vi "MQTT_Connect.vi"(5 "Connect Meta":T5={"QoS"=enum."At most once", "DUP"=FALSE, "Retain"=TRUE, "Keep Alive (sec)"=60}, 6 "Client ID":string="LabVIEW_MQTT_Client", 7 "Connect Flags":T8, 8 "error in (no error)":errorcluster, 9 "Will Info":T6={"Will message"="Last Will", "Will Topic"="Will Topic"}, 10 "User Info":T7={"User Name"="User", "Password"="password"}, 11 "MQTT Broker":cluster{"address (IP)":string, "port":u16}={"address (IP)"="broker.mqttdashboard.com", "port"=1883}) -> (0 "error out":errorcluster, 2 "Connection Status":T1=enum."Connection refused: not authorized", 3 "connection ID out":refnum<k5>)   [LabVIEW 2025, in "MQTT_Functions.lvlib"]
doc: "Connects to an MQTT broker server with required settings. \n\n© 2015 - daq.io, LLC - Peter Adelhardt"
uses:
  MQTT_Functions.lvlib
  Controls/Connect_Flags.ctl
  Controls/QoS.ctl
  Controls/User_Info.ctl
  Controls/Will_Info.ctl
  Controls/DUP_Flag.ctl
  Controls/Retain_Flag.ctl
  Controls/Connection_Return_Codes.ctl
  Controls/Conn_FGV_Cmds.ctl
  Controls/Conn_Stat_FGV_Cmds.ctl
  Controls/MessageType.ctl
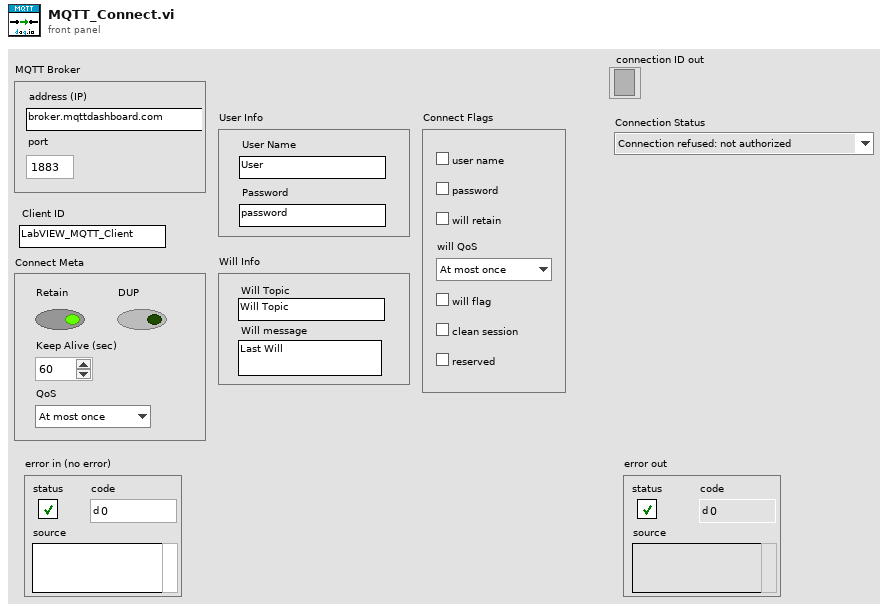
[diagram p1: front panel]
types:
  T1 = typedef "MQTT_Functions.lvlib/Connection_Return_Codes.ctl" = enum16{"Connection accepted", "Connection refused: unacceptable protocol version", "Connection refused: identifier rejected", "Connection refused: Server unavailable", "Connection refused: bad user name or password", "Connection refused: not authorized"}
  T2 = typedef "MQTT_Functions.lvlib/QoS.ctl" = enum8{"At most once", "At least once", "Exactly once", "Reserved"}
  T3 = typedef "MQTT_Functions.lvlib/DUP_Flag.ctl" = bool
  T4 = typedef "MQTT_Functions.lvlib/Retain_Flag.ctl" = bool
  T5 = cluster{"QoS":T2, "DUP":T3, "Retain":T4, "Keep Alive (sec)":u16}
  T6 = typedef "MQTT_Functions.lvlib/Will_Info.ctl" = cluster{"Will message":string, "Will Topic":string}
  T7 = typedef "MQTT_Functions.lvlib/User_Info.ctl" = cluster{"User Name":string, "Password":string}
  T8 = typedef "MQTT_Functions.lvlib/Connect_Flags.ctl" = cluster{"user name":bool, "password":bool, "will retain":bool, "will flag":bool, "clean session":bool, "reserved":bool, "will QoS":T2}
  T9 = typedef "MQTT_Functions.lvlib/Conn_Stat_FGV_Cmds.ctl" = enum16{"Get", "Set"}
  T10 = typedef "MQTT_Functions.lvlib/Conn_FGV_Cmds.ctl" = enum16{"Get", "Set", "Delete"}
  T11 = typedef "MQTT_Functions.lvlib/MessageType.ctl" = enum32{"Reserved", "CONNECT", "CONNACK", "PUBLISH", "PUBACK", "PUBREC", "PUBREL", "PUBCOMP", "SUBSCRIBE", "SUBACK", "UNSUBSCRIBE", "UNSUBACK", "PINGREQ", "PINGRESP", "DISCONNECT", "Reserved2"}
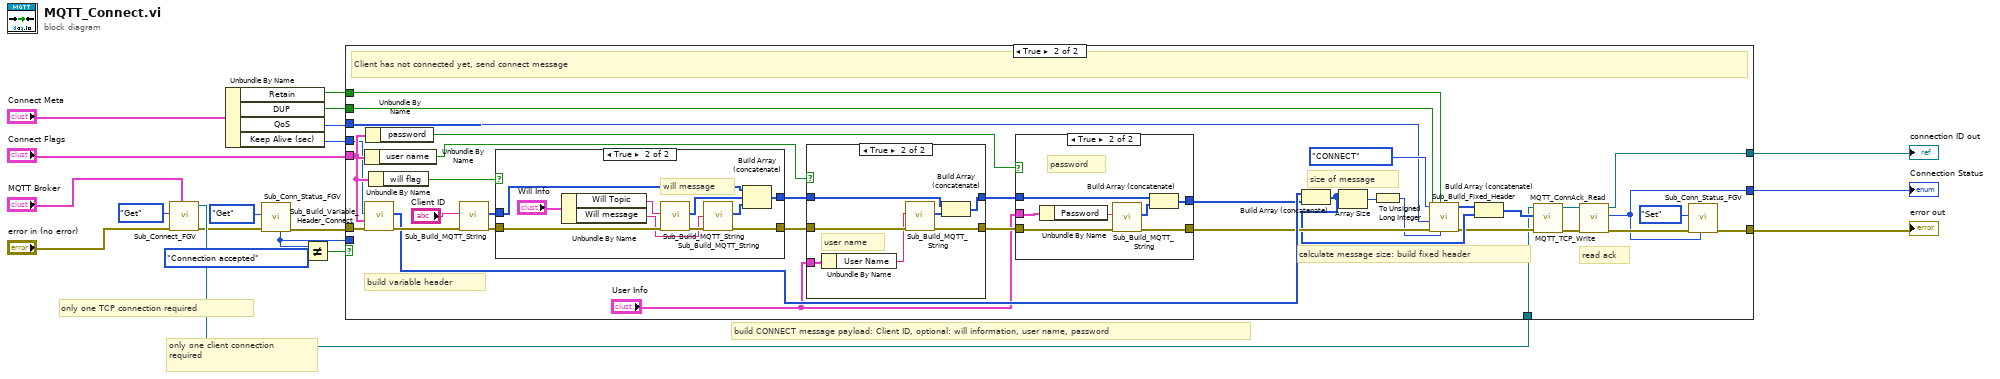
[diagram p0: block diagram]
diagram:
  # "only one client connection\nrequired"
  # "only one TCP connection required"
  # "build CONNECT message payload: Client ID, optional: will information, user name, password"
  n1 = call "Sub_Connect_FGV.vi"("MQTT Broker"="MQTT Broker", "error in"="error in (no error)", "Command"=Conn_FGV_Cmds."Get") -> ("error out"=w5:errorcluster, "MQTT ref out"=w12:refnum<k5>)  [unwired: 7 in]
  n2 = Unbundle By Name("Connect Meta") -> ("Retain"=w17:T4, "DUP"=w16:T3, "QoS"=w15:T2, "Keep Alive (sec)"=w14:u16)
  n3 = call "Sub_Conn_Status_FGV.vi"("error in"=w5, "Command"=Conn_Stat_FGV_Cmds."Get") -> ("error out"=w2:errorcluster, "Connection Status out"=w1:T1)  [unwired: 8 in]
  n4 = Not Equal?(x=w1, y=Connection_Return_Codes."Connection accepted") -> (x != y?=w3:bool)
  n5 = case shown="True" w3 {
    tunnel: "Connect Flags" -> [_ w52]
    tunnel: w17 -> [_ w38]
    tunnel: w16 -> [_ w37]
    tunnel: w15 -> [_ w36]
    tunnel: w14 -> [_ w35]
    tunnel: w2 -> [w22 w29]
    tunnel: w12 -> [w20 w28]
    tunnel: [w22 w24] -> w9
    tunnel: [w21 w23] -> w8
    tunnel: [w20 w27] -> w7
    tunnel: w1 -> [w21 _]
    frame False {
      # "client is already connected"
    }
    frame True {
      # "read ack"
      # "calculate message size: build fixed header"
      # "build variable header"
      # "size of message"
      # "Client has not connected yet, send connect message"
      n6 = Unbundle By Name(w52) -> ("user name"=w51:bool)
      n7 = call "Sub_Build_Variable_Header_Connect.vi"("error in (no error)"=w29, "Connect Flags"=w52, "Keep Alive (sec)"=w35) -> ("error out"=w57:errorcluster, "Variable Header"=w48:u8[])  [unwired: 7 in]
      n8 = Unbundle By Name(w52) -> ("password"=w50:bool)
      n9 = Unbundle By Name(w52) -> ("will flag"=w49:bool)
      n10 = call "Sub_Build_MQTT_String.vi"("error in (no error)"=w57, "String to be encoded"="Client ID") -> ("error out"=w53:errorcluster, "UTF8 Byte Array"=w56:u8[])  [unwired: 8 in]
      n11 = case shown="True" w49 {
        tunnel: w56 -> [w78 w86]
        tunnel: [w78 w87] -> w55
        tunnel: w53 -> [w77 w85]
        tunnel: [w77 w82] -> w46
        frame False {
        }
        frame True {
          # "will message"
          n12 = Unbundle By Name("Will Info") -> ("Will Topic"=w80:string, "Will message"=w79:string)
          n13 = call "Sub_Build_MQTT_String.vi"("error in (no error)"=w85, "String to be encoded"=w80) -> ("error out"=w84:errorcluster, "UTF8 Byte Array"=w83:u8[])  [unwired: 8 in]
          n14 = call "Sub_Build_MQTT_String.vi"("error in (no error)"=w84, "String to be encoded"=w79) -> ("error out"=w82:errorcluster, "UTF8 Byte Array"=w88:u8[])  [unwired: 8 in]
          n15 = Build Array (concatenate)(w86, w83, w88) -> (w87:u8[])
        }
      }
      n16 = case shown="True" w51 {
        tunnel: w55 -> [w69 w75]
        tunnel: [w69 w74] -> w54
        tunnel: [w68 w73] -> w47
        tunnel: w46 -> [w68 w72]
        tunnel: "User Info" -> [_ w71]
        frame False {
        }
        frame True {
          # "user name"
          n17 = Unbundle By Name(w71) -> ("User Name"=w70:string)
          n18 = call "Sub_Build_MQTT_String.vi"("error in (no error)"=w72, "String to be encoded"=w70) -> ("error out"=w73:errorcluster, "UTF8 Byte Array"=w76:u8[])  [unwired: 8 in]
          n19 = Build Array (concatenate)(w75, w76) -> (w74:u8[])
        }
      }
      n20 = case shown="True" w50 {
        tunnel: w54 -> [w60 w66]
        tunnel: [w60 w65] -> w44
        tunnel: w47 -> [w59 w64]
        tunnel: [w59 w63] -> w45
        tunnel: "User Info" -> [_ w62]
        frame False {
        }
        frame True {
          # "password"
          n21 = Unbundle By Name(w62) -> ("Password"=w61:string)
          n22 = call "Sub_Build_MQTT_String.vi"("error in (no error)"=w64, "String to be encoded"=w61) -> ("error out"=w63:errorcluster, "UTF8 Byte Array"=w67:u8[])  [unwired: 8 in]
          n23 = Build Array (concatenate)(w66, w67) -> (w65:u8[])
        }
      }
      n24 = Build Array (concatenate)(w48, w44) -> (w43:u8[])
      n25 = Array Size(array=w43) -> (size(s)=w41:i32)
      n26 = To Unsigned Long Integer(number=w41) -> (unsigned 32bit integer=w40:u32)
      n27 = call "Sub_Build_Fixed_Header.vi"("Remaining Length"=w40, "Retain"=w38, "error in (no error)"=w45, "QoS"=w36, "DUP"=w37, "MessageType"=MessageType."CONNECT") -> ("error out"=w33:errorcluster, "Fixed Header"=w42:u8[])  [unwired: 4 in]
      n28 = Build Array (concatenate)(w42, w43) -> (w32:u8[])
      n29 = call "MQTT_TCP_Write.vi"("error in (no error)"=w33, "data in"=w32, "connection ID"=w28) -> ("error out"=w31:errorcluster, "connection ID out"=w30:refnum<k5>)  [unwired: 6 in, 1 out]
      n30 = call "MQTT_ConnAck_Read.vi"("error in (no error)"=w31, "connection ID"=w30) -> ("error out"=w26:errorcluster, "Connection Status"=w23:T1, "connection ID out"=w27:refnum<k5>)  [unwired: 5 in, 2 out]
      n31 = call "Sub_Conn_Status_FGV.vi"("Connection Status in"=w23, "error in"=w26, "Command"=Conn_Stat_FGV_Cmds."Set") -> ("error out"=w24:errorcluster)  [unwired: 7 in, 1 out]
    }
  }
  "error out" <- w9
  "connection ID out" <- w7
  "Connection Status" <- w8
